vi "Send.vi"(8 "error in (no error)":errorcluster, 10 "data":string, 11 "Serial Base in":refnum<class "Serial Base.lvclass">) -> (0 "error out":errorcluster, 2 "bytes count":u32, 3 "Serial Base out":refnum<class "Serial Base.lvclass">)   [LabVIEW 2014, in "Serial Base.lvclass"]
doc: "<b>Description</b>\nSend data string into the serial port buffer.\n------------------------------------------------\n<b>data</b>: contains the data to be sent to the device. \n\n<b>bytes count</b>: return count contains the actual number of bytes written."
uses:
  Serial Base.lvclass
  Serial Base.lvclass/Serial Base.ctl
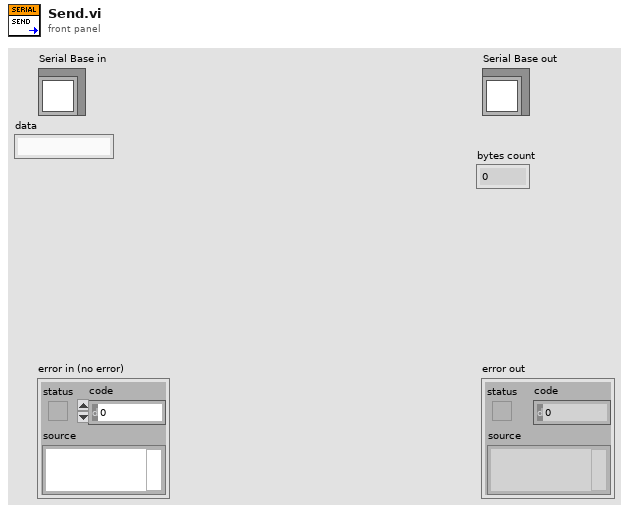
[diagram p1: front panel]
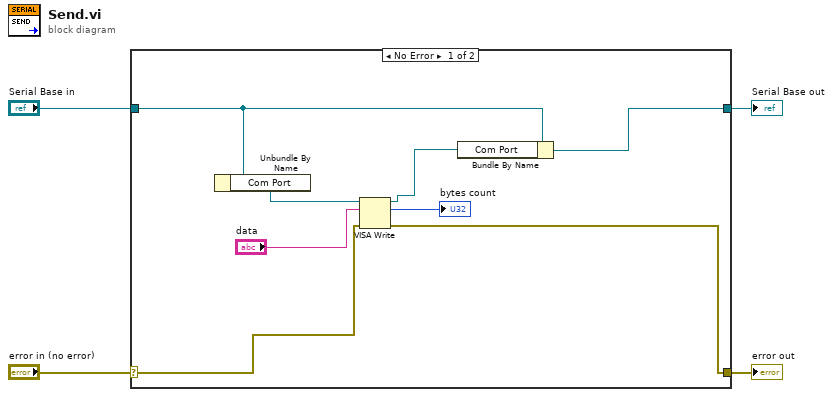
[diagram p0: block diagram]
diagram:
  n1 = case shown="No Error" "error in (no error)" {
    selector: "error in (no error)" -> [w10 w14]
    tunnel: [w9 w14] -> w3
    tunnel: [w6 w13] -> w1
    tunnel: "Serial Base in" -> [w7 w13]
    frame No Error {
      n2 = Unbundle By Name(w7) -> ("Com Port"=w12:refnum<visa-resource-name>)
      n3 = VISA Write(VISA resource name=w12, write buffer="data", error in (no error)=w10) -> (VISA resource name out=w8:refnum<visa-resource-name>, return count=→"bytes count":u32, error out=w9:errorcluster)
      n4 = Bundle By Name(cluster=w7, "Com Port"=w8) -> (w6:refnum<class "Serial Base.lvclass">)
    }
    frame Error {
    }
  }
  "error out" <- w3
  "Serial Base out" <- w1
